vi "Write Item Names.vi"(8 "error in (no error)":errorcluster, 10 "ItemNames":string[][](array[string]), 11 "DataGrid.lvclass in":refnum<class "DataGrid.lvclass">) -> (0 "error out":errorcluster, 3 "DataGrid.lvclass out":refnum<class "DataGrid.lvclass">)   [LabVIEW 2017, in "DataGrid.lvclass"]
uses:
  DataGrid.lvclass
  <vilib>/QSI/QControls/QControl Classes/MulticolumnListbox/MulticolumnListbox.lvclass
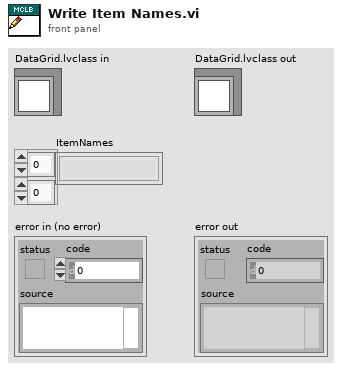
[diagram p1: front panel]
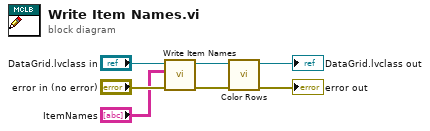
[diagram p0: block diagram]
diagram:
  n1 = call-parent "Write Item Names.vi"("error in (no error)"="error in (no error)", "ItemNames"="ItemNames", "MulticolumnListbox.lvclass in"="DataGrid.lvclass in") -> ("error out"=w2:errorcluster, "MulticolumnListbox.lvclass out"=w4:refnum<class "DataGrid.lvclass">)  [unwired: 7 in]
  n2 = call "Color Rows.vi"("error in (no error)"=w2, "DataGrid in"=w4) -> ("error out"=→"error out":errorcluster, "DataGrid out"=→"DataGrid.lvclass out":refnum<class "DataGrid.lvclass">)  [unwired: 8 in]
